vi "A-C.vi"(0 "KNR in":T1, 3 "error in (no error)":errorcluster) -> (7 "KNR out":T1, 10 "error out":errorcluster)   [LabVIEW 2013]
uses:
  <userlib>/KNR OS 3.0 LabVIEW Toolkit/Type Definition/KNR3 Reference.ctl
  <userlib>/_FPGA Interface Advanced Tools/FPGA Interface Base/FPGA Interface Base.lvclass
  <userlib>/KNR OS 3.0 LabVIEW Toolkit/Type Definition/Resource.ctl
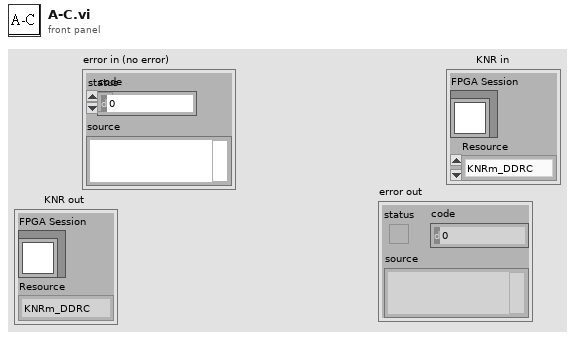
[diagram p1: front panel]
types:
  T1 = typedef "KNR3 Reference.ctl" = cluster{"FPGA Session":refnum<class "FPGA Interface Base.lvclass">, "Resource":T2}
  T2 = typedef "Resource.ctl" = enum16{"KNRm_DDRC", "KNRm_DDDD", "KNRm_DDDR", "KNRm_DDDC", "KNR"}
  T3 = cluster{"Mode":enum16{"FRWD", "TURFIX", "TURNOF", "CIRCULAR"}, "Dir":enum16{"Left", "Right"}, "Pcmd":dbl, "Vcmd":dbl, "X":dbl, "Y":dbl}
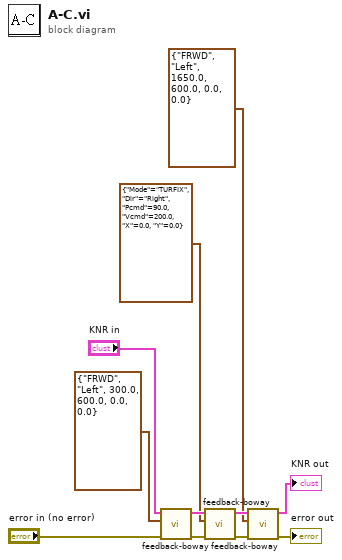
[diagram p0: block diagram]
diagram:
  n1 = call "feedback-boway.vi"("error in (no error)"="error in (no error)", "Move"=T3 {"Mode"=enum."FRWD", "Dir"=enum."Left", "Pcmd"=300.0, "Vcmd"=600.0, "X"=0.0, "Y"=0.0}, "KNR in"="KNR in") -> ("error out"=w6:errorcluster, "KNR out"=w8:T1)  [unwired: 6 in, 1 out]
  n2 = call "feedback-boway.vi"("error in (no error)"=w6, "Move"=T3 {"Mode"=enum."TURFIX", "Dir"=enum."Right", "Pcmd"=90.0, "Vcmd"=200.0, "X"=0.0, "Y"=0.0}, "KNR in"=w8) -> ("error out"=w3:errorcluster, "KNR out"=w7:T1)  [unwired: 6 in, 1 out]
  n3 = call "feedback-boway.vi"("error in (no error)"=w3, "Move"=T3 {"Mode"=enum."FRWD", "Dir"=enum."Left", "Pcmd"=1650.0, "Vcmd"=600.0, "X"=0.0, "Y"=0.0}, "KNR in"=w7) -> ("error out"=→"error out":errorcluster, "KNR out"=→"KNR out":T1)  [unwired: 6 in, 1 out]
